vi "Version CompareTo.vi"(10 "version 2":string, 11 "version 1":string) -> (3 "comparison":i32)   [LabVIEW 2015, in "Chassis TimeSync System Explorer.lvlib"]
uses:
  Chassis TimeSync System Explorer.lvlib
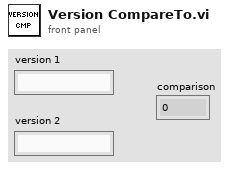
[diagram p1: front panel]
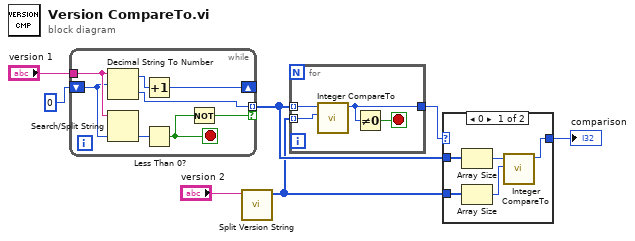
[diagram p0: block diagram]
diagram:
  n1 = while {
    tunnel: "version 1" -> [w14]
    shift-right: [w10] -> _
    shift-left: 0 -> [w13]
    tunnel: [w15] -> w3 mode=indexing if=w9
    stop <- w8 stop-if-true
    n2 = Decimal String To Number(string=w14, offset=w13) -> (offset past number=w11:i32, number=w15:i32)  [unwired: 1 in]
    n3 = Search/Split String(string=w14, offset (0)=w13) -> (offset of match=w12:i32)  [unwired: 1 in, 2 out]
    n4 = Increment(x=w11) -> (x+1=w10:i32)
    n5 = Less Than 0?(x=w12) -> (x < 0?=w8:bool)
    n6 = Not(x=w8) -> (.not. x?=w9:bool)
  }
  n7 = call "Split Version String.vi"("version"="version 2") -> ("split version"=w2:i32[])  [unwired: 10 in]
  n8 = for {
    tunnel: w3 -> [w19] mode=indexing
    tunnel: w2 -> [w18] mode=indexing
    tunnel: [w17] -> w4
    stop <- w16 stop-if-true
    n9 = call "Integer CompareTo.vi"("input 2"=w18, "input 1"=w19) -> ("comparison"=w17:i32)  [unwired: 9 in]
    n10 = Not Equal To 0?(x=w17) -> (x != 0?=w16:bool)
  }
  n11 = case shown="0" w4 {
    selector: w4 -> [_ w25]
    tunnel: [w20 w25] -> w1
    tunnel: w3 -> [w24 _]
    tunnel: w2 -> [w23 _]
    frame 0 {
      n12 = Array Size(array=w24) -> (size(s)=w22:i32)
      n13 = Array Size(array=w23) -> (size(s)=w21:i32)
      n14 = call "Integer CompareTo.vi"("input 2"=w21, "input 1"=w22) -> ("comparison"=w20:i32)  [unwired: 9 in]
    }
    frame Default {
    }
  }
  "comparison" <- w1
